vi "Init Device.vi"(7 "Layout Ref":refnum<vi>, 8 "error in (no error)":errorcluster, 10 "Chan# Array":i32[](array[numeric]), 11 "Arduino in":refnum<class "Arduino.lvclass">) -> (0 "error out":errorcluster, 3 "Arduino out":refnum<class "Arduino.lvclass">)   [LabVIEW 2013, in "Arduino.lvclass"]
doc: "Initialize the correct columns and their default appearance.\nUse the front panel to change default appearance of the device in the Add/Manage devices.\n\nOpen a specific device implementation for details."
uses:
  Arduino.lvclass
  TypeDefs/ColumnAppearCluster.ctl
  ColumnVIs/Column/Column.lvclass
panel:
  in  "Command Arguments":T1={"Column Name"="", "Width"=30, "Bkgd"=[16448250], "Text"=[0]}
  # "Open a specific devices override of this VI for implementation."
  # "Intended functionality:\n------------------------\nPlace controls here for Device programmer OR advanced user to configure\ntypical layout in the table.\n\nDisplay Info.vi (called on add/manage device) will be where typical user can fine tune."
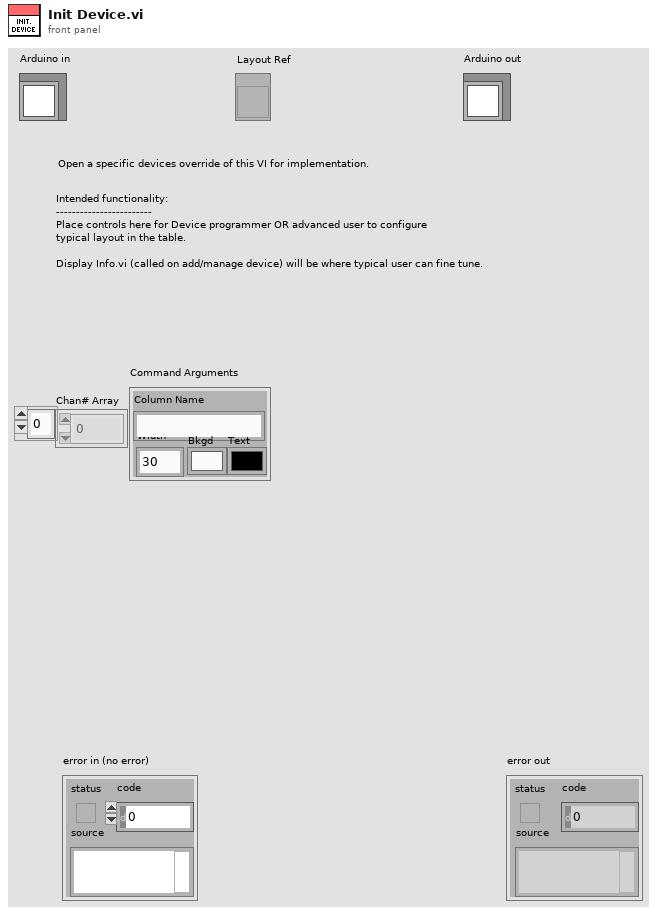
[diagram p1: front panel]
types:
  T1 = typedef "ColumnAppearCluster.ctl" = cluster{"Column Name":string, "Width":u32, "Bkgd":u32[], "Text":u32[]}
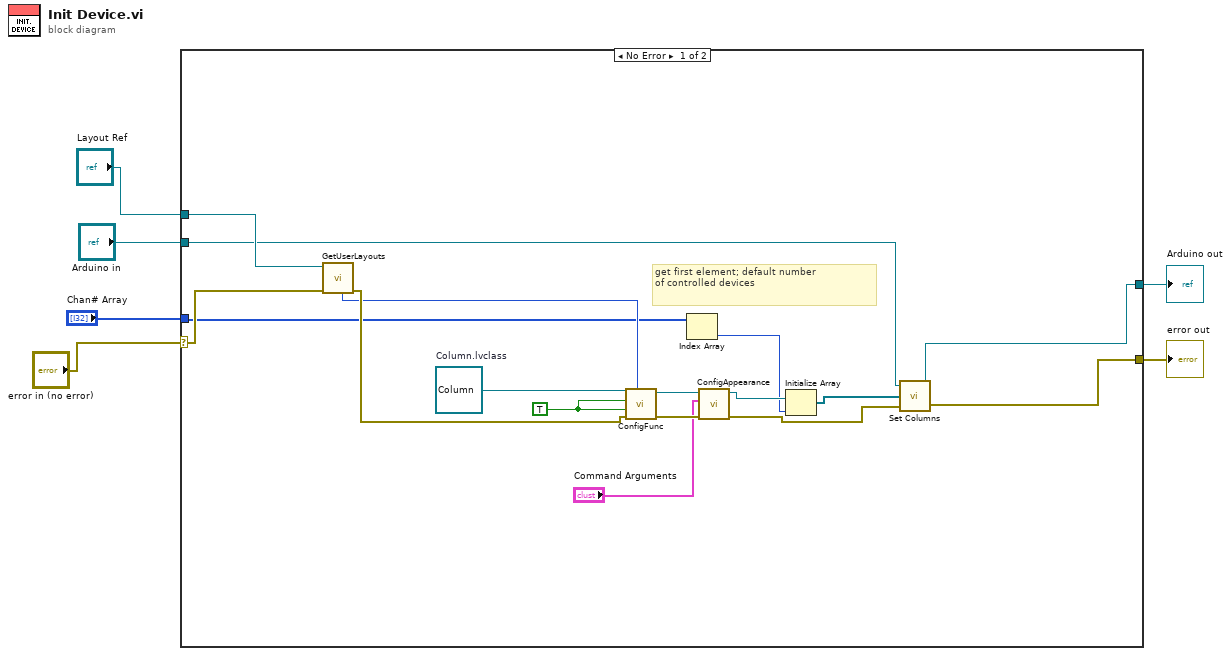
[diagram p0: block diagram]
diagram:
  n1 = case shown="No Error" "error in (no error)" {
    selector: "error in (no error)" -> [w23 w25]
    tunnel: [w8 w25] -> w5
    tunnel: "Arduino in" -> [w10 w24]
    tunnel: [w9 w24] -> w3
    tunnel: "Layout Ref" -> [w22 _]
    tunnel: "Chan# Array" -> [w13 _]
    frame No Error {
      w20 = refnum<class "Column.lvclass"> refnum  # Column.lvclass
      w21 = TRUE
      # "get first element; default number\nof controlled devices"
      n2 = call "GetUserLayouts.vi"("error in (no error)"=w23, "Layout Ring Refnum"=w22) -> ("error out"=w18:errorcluster, "Num User Layouts"=w15:i32)  [unwired: 5 in, 3 out]
      n3 = call "ConfigFunc.vi"("Num Layouts (ignored)"=w15, "error in (no error)"=w18, "isVariable? (True)"=w21, "Disableable? (True)"=w21, "Column in"=w20) -> ("error out"=w17:errorcluster, "Column out"=w19:refnum<class "Column.lvclass">)  [unwired: 5 in]
      n4 = Index Array(array=w13) -> (element=w12:i32)  [unwired: 1 in]
      n5 = call "ConfigAppearance.vi"("error in (no error)"=w17, "Column Appearance"="Command Arguments", "Column in"=w19) -> ("error out"=w7:errorcluster, "Column out"=w14:refnum<class "Column.lvclass">)  [unwired: 7 in]
      n6 = Initialize Array(w14, w12) -> (w11:refnum<class "Column.lvclass">[])
      n7 = call-dynamic "Set Columns.vi"("error in (no error)"=w7, "Columns"=w11, "Device in"=w10) -> ("error out"=w8:errorcluster, "Device out"=w9:refnum<class "Arduino.lvclass">)  [unwired: 1 in]
    }
    frame Error {
    }
  }
  "error out" <- w5
  "Arduino out" <- w3
